vi "Check Warn,NS,EStop Thresholds.vi"(8 "error in (no error)":errorcluster, 10 "Current Vals":T6, 11 "[[APU Sensor Info]]":string[][](array[string])) -> (0 "error out":errorcluster, 3 "[Tags and Alerts]":T1[](array[typedef]))   [LabVIEW 2018, in "RT - Analysis.lvlib"]
uses:
  RT - Analysis.lvlib
  Top Level/Shared Controls/Post-Analysis Data.ctl
  Top Level/Shared Controls/Calculated Data.ctl
  Private Controls/Parsed Data Arrays.ctl
  Top Level/Shared Controls/Parsed Tag Cluster.ctl
  Public Controls/Alert Data.ctl
  <vilib>/dlg_ctls.llb/Space Constant.vi
  Check Tag WarnNSEstop Threshold.vi
  <userlib>/_OpenG.lib/lvdata/lvdata.llb/Array Size(s)__ogtk.vi
  <userlib>/_OpenG.lib/lvdata/lvdata.llb/Array to Array of VData__ogtk.vi
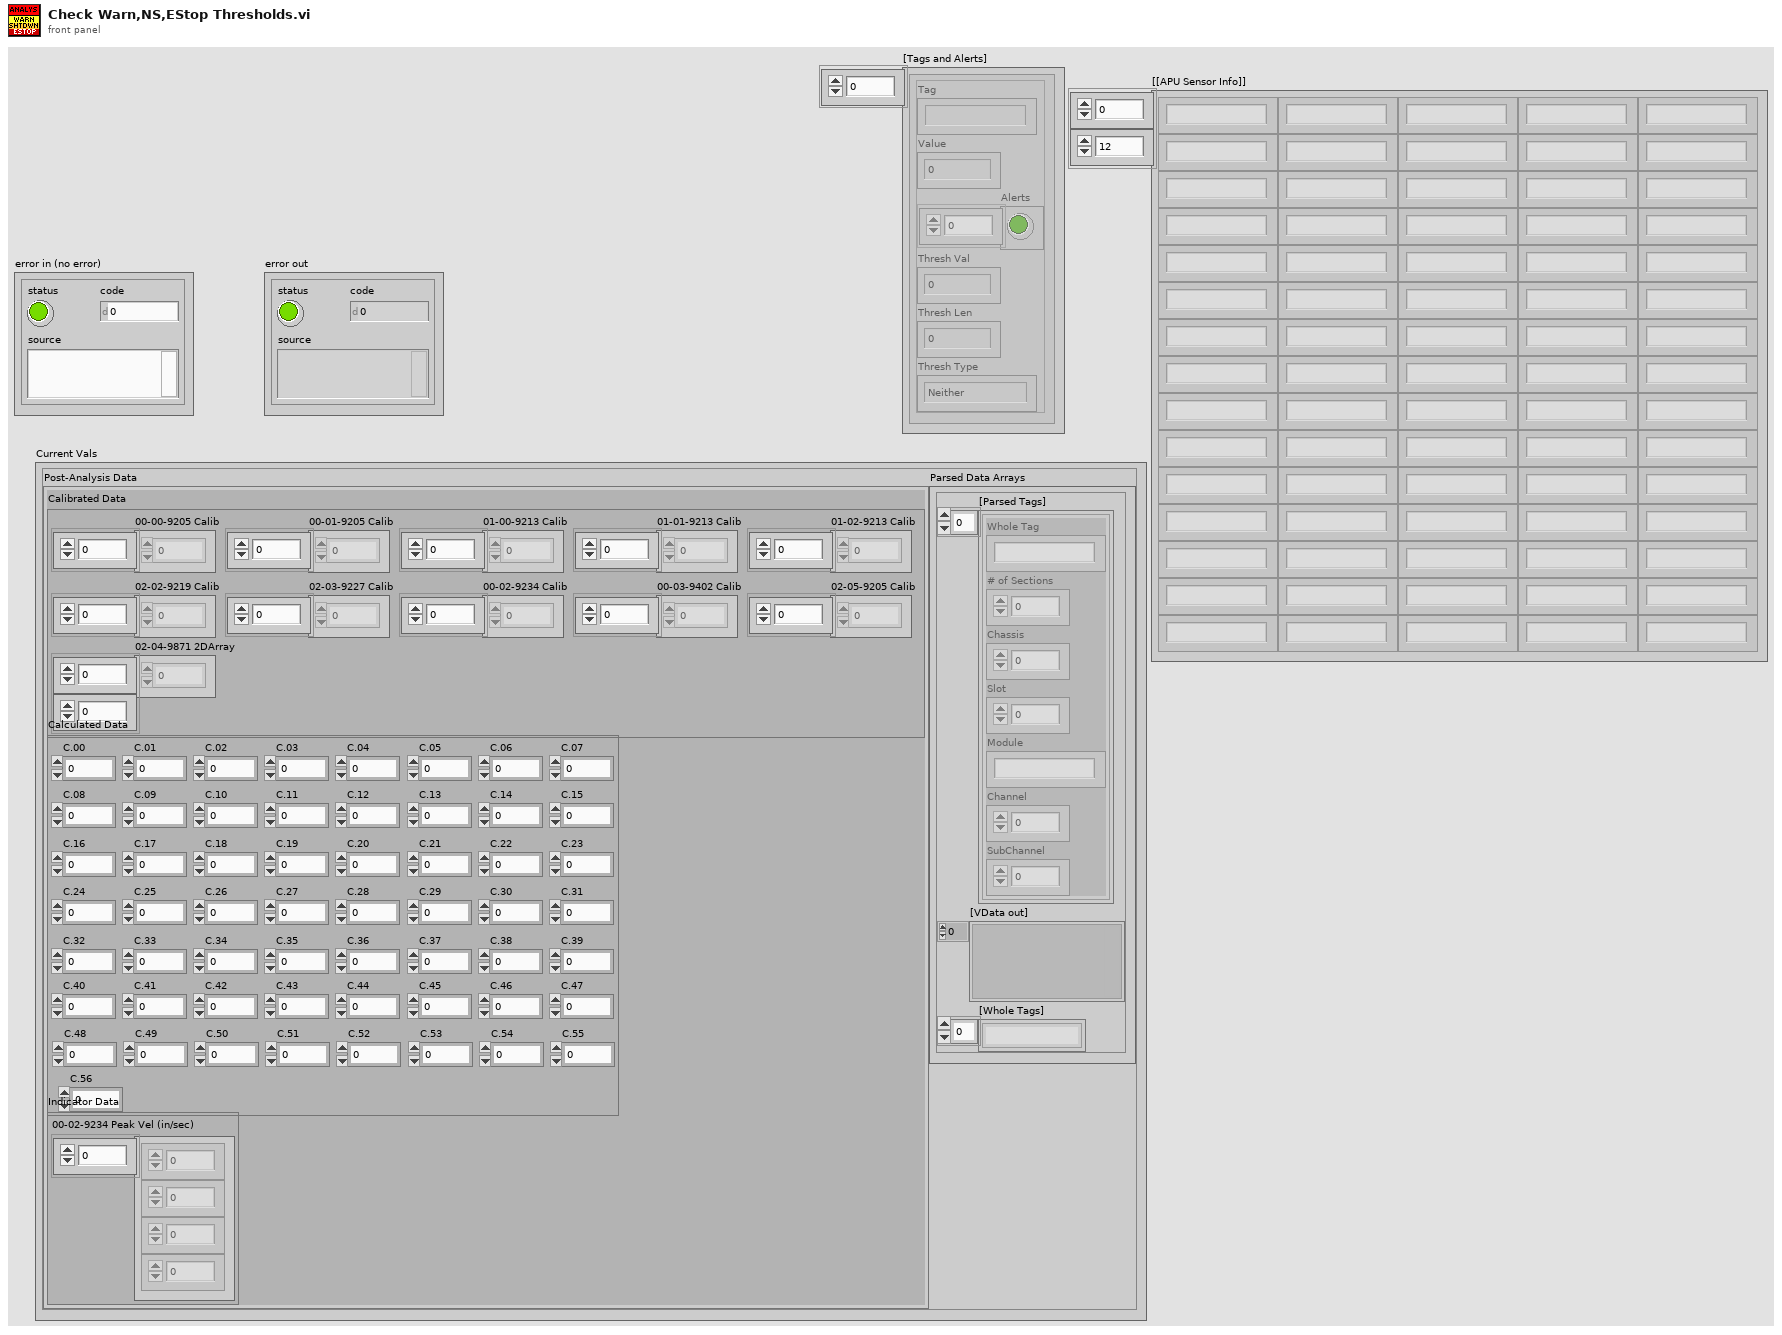
[diagram p1: front panel]
types:
  T1 = typedef "RT - Analysis.lvlib/Alert Data.ctl" = cluster{"Tag":string, "Value":dbl, "Alerts":bool[], "Thresh Val":dbl, "Thresh Len":dbl, "Thresh Type":enum16{"Neither", "Max", "Min"}}
  T2 = typedef "Post-Analysis Data.ctl" = cluster{"Calibrated Data":cluster{"00-00-9205 Calib":dbl[], "00-01-9205 Calib":dbl[], "01-00-9213 Calib":dbl[], "01-01-9213 Calib":dbl[], "01-02-9213 Calib":dbl[], "02-02-9219 Calib":dbl[], "02-03-9227 Calib":dbl[], "00-02-9234 Calib":dbl[], "00-03-9402 Calib":dbl[], "02-05-9205 Calib":dbl[], "02-04-9871 2DArray":dbl[][]}, "Calculated Data":T3, "Indicator Data":cluster{"00-02-9234 Peak Vel (in/sec)":dbl[]}}
  T3 = typedef "Calculated Data.ctl" = cluster{"C.00":dbl, "C.01":dbl, "C.02":dbl, "C.03":dbl, "C.04":dbl, "C.05":dbl, "C.06":dbl, "C.07":dbl, "C.08":dbl, "C.09":dbl, "C.10":dbl, "C.11":dbl, "C.12":dbl, "C.13":dbl, "C.14":dbl, "C.15":dbl, "C.16":dbl, "C.17":dbl, "C.18":dbl, "C.19":dbl, "C.20":dbl, "C.21":dbl, "C.22":dbl, "C.23":dbl, "C.24":dbl, "C.25":dbl, "C.26":dbl, "C.27":dbl, "C.28":dbl, "C.29":dbl, "C.30":dbl, "C.31":dbl, "C.32":dbl, "C.33":dbl, "C.34":dbl, "C.35":dbl, "C.36":dbl, "C.37":dbl, "C.38":dbl, "C.39":dbl, "C.40":dbl, "C.41":dbl, "C.42":dbl, "C.43":dbl, "C.44":dbl, "C.45":dbl, "C.46":dbl, "C.47":dbl, "C.48":dbl, "C.49":dbl, "C.50":dbl, "C.51":dbl, "C.52":dbl, "C.53":dbl, "C.54":dbl, "C.55":dbl, "C.56":dbl}
  T4 = typedef "RT - Analysis.lvlib/Parsed Data Arrays.ctl" = cluster{"[Parsed Tags]":T5[], "[VData out]":variant[], "[Whole Tags]":string[]}
  T5 = typedef "Parsed Tag Cluster.ctl" = cluster{"Whole Tag":string, "# of Sections":u8, "Chassis":u8, "Slot":u8, "Module":string, "Channel":u8, "SubChannel":u8}
  T6 = cluster{"Post-Analysis Data":T2, "Parsed Data Arrays":T4}
  T7 = cluster{"Warn Timer Start":u32, "NS Timer Start":u32, "Estop Timer Start":u32}
  T8 = cluster{"Warn Timer Start":u32, "NS Timer Start":u32, "Estop Timer Start":u32}[]
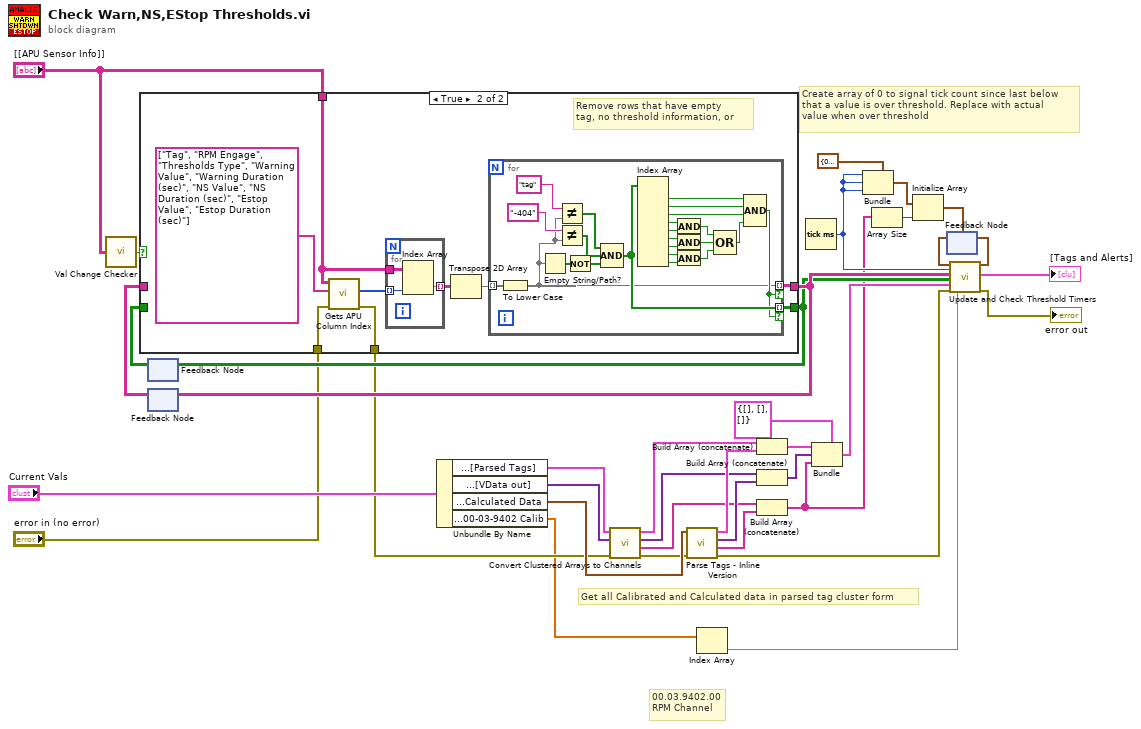
[diagram p0: block diagram]
diagram:
  # "00.03.9402.00\nRPM Channel"
  # "Get all Calibrated and Calculated data in parsed tag cluster form"
  # "Create array of 0 to signal tick count since last below\nthat a value is over threshold. Replace with actual\nvalue when over threshold"
  n1 = call "Val Change Checker.vi"("Current Value in"="[[APU Sensor Info]]") -> ("Value Change?"=w1:bool)
  n2 = feedback #1() -> (w14:bool[][])  [unwired: 1 in]
  n3 = feedback #2() -> (w27:string[][])  [unwired: 1 in]
  n4 = case shown="True" w1 {
    tunnel: [w38 w45] -> w11
    tunnel: "error in (no error)" -> [w38 w44]
    tunnel: "[[APU Sensor Info]]" -> [_ w43]
    tunnel: [w39 w41] -> w28
    tunnel: w27 -> [w39 _]
    tunnel: [w37 w40] -> w15
    tunnel: w14 -> [w37 _]
    frame False {
      # "Unless APU Sensor Info changes, pass previous array"
    }
    frame True {
      # "Remove rows that have empty\ntag, no threshold information, or"
      n5 = call "Gets APU Column Index.vi"("error in (no error)"=w44, "[Column Names]"=string[] ["Tag", "RPM Engage", "Thresholds Type", "Warning Value", "Warning Duration (sec)", "NS Value", "NS Duration (sec)", "Estop Value", "Estop Duration (sec)"], "[[Array of Info]]"=w43) -> ("error out"=w45:errorcluster, "[Col Indices]"=w47:i32[])  [unwired: 4 in, 3 out]
      n6 = for {
        tunnel: w43 -> [w74]
        tunnel: w47 -> [w73] mode=indexing
        tunnel: [w72] -> w48 mode=indexing
        n7 = Index Array(array=w74, index (col)=w73) -> (element=w72:string[])  [unwired: 1 in]
      }
      n8 = Transpose 2D Array(2D array=w48) -> (transposed array=w42:string[][])
      n9 = for {
        tunnel: w42 -> [w66] mode=indexing
        tunnel: [w50] -> w41 mode=indexing if=w51
        tunnel: [w52] -> w40 mode=indexing if=w51
        n10 = To Lower Case(string=w66) -> (all lower case string=w50:string[])
        n11 = Empty String/Path?(string/path=w50) -> (empty?=w71:bool[])
        n12 = Not Equal?(x="tag" ("String"), y=w50) -> (x != y?=w67:bool[])
        n13 = Not Equal?(x="-404" ("String"), y=w50) -> (x != y?=w69:bool[])
        n14 = Not(x=w71) -> (.not. x?=w70:bool[])
        n15 = Compound Arithmetic op=AND(w67, w69, w70) -> (w52:bool[])
        n16 = Index Array(array=w52) -> (element #1=w49:bool, element #2=w64:bool, element #3=w63:bool, element #4=w62:bool, element #5=w61:bool, element #6=w60:bool, element #7=w57:bool, element #8=w59:bool, element #9=w58:bool)  [unwired: 9 in]
        n17 = And(x=w62, y=w61) -> (x .and. y?=w56:bool)
        n18 = And(x=w60, y=w57) -> (x .and. y?=w55:bool)
        n19 = And(x=w59, y=w58) -> (x .and. y?=w54:bool)
        n20 = Compound Arithmetic op=OR(w56, w55, w54) -> (w53:bool)
        n21 = Compound Arithmetic op=AND(w49, w64, w63, w53) -> (w51:bool)
      }
    }
  }
  n22 = feedback-in #1(w15) -> ()
  n23 = feedback-in #2(w28) -> ()
  n24 = Unbundle By Name("Current Vals") -> ("Parsed Data Arrays.[Parsed Tags]"=w8:T5[], "Parsed Data Arrays.[VData out]"=w7:variant[], "Post-Analysis Data.Calculated Data"=w21:T3, "Post-Analysis Data.Calibrated Data.00-03-9402 Calib"=w9:dbl[])
  n25 = call "Convert Clustered Arrays to Channels.vi"("error in (no error)"=w11, "[VData out]"=w7, "[Parsed Tags]"=w8) -> ("error out"=w18:errorcluster, "[Whole Tags]"=w19:string[], "[VData out]"=w4:variant[], "[Parsed Tags]"=w20:T5[])  [unwired: 5 in]
  n26 = call "Parse Tags - Inline Version.vi"("error in (no error)"=w18, "Cluster of Controls"=w21) -> ("error out"=w13:errorcluster, "[Whole Tags]"=w34:string[], "[VData out]"=w35:variant[], "[Parsed Tags]"=w36:T5[])  [unwired: 6 in]
  n27 = Index Array(array=w9) -> (element=w3:dbl)  [unwired: 1 in]
  n28 = Build Array (concatenate)(w20, w36) -> (w33:T5[])
  n29 = Build Array (concatenate)(w4, w35) -> (w32:variant[])
  n30 = Build Array (concatenate)(w19, w34) -> (w6:string[])
  n31 = Tick Count (ms)() -> (millisecond timer value=w24:u32)
  n32 = Bundle(cluster=T4 {"[Parsed Tags]"=[], "[VData out]"=[], "[Whole Tags]"=[]} ("Parsed Data Arrays"), "[Parsed Tags]"=w33, "[VData out]"=w32, "[Whole Tags]"=w6) -> (w31:T4)
  n33 = Bundle(cluster=T7 {"Warn Timer Start"=0, "NS Timer Start"=0, "Estop Timer Start"=0} ("Timers"), "Warn Timer Start"=w24, "NS Timer Start"=w24, "Estop Timer Start"=w24) -> (w23:T7)
  n34 = Array Size(array=w6) -> (size(s)=w30:i32)
  n35 = Initialize Array(w23, w30) -> (w29:T8)
  n36 = feedback #3(w29) -> (w26:T8)
  n37 = call "Update and Check Threshold Timers.vi"("[Prev Threshold Timers]"=w26, "Current Tick Count"=w24, "[Threshold Settings]"=w28, "[Threshold Settings Present Bools]"=w15, "[Parsed Controls]"=w31, "error in (no error)"=w13, "Current RPM"=w3) -> ("[New Threshold Timers]"=w25:T8, "[Alerts] out"=→"[Tags and Alerts]":T1[], "error out"=→"error out":errorcluster)  [unwired: 10 in]
  n38 = feedback-in #3(w25) -> ()
